vi "Error Query.vi"(8 "error in (no error)":errorcluster, 11 "VISA resource name":refnum<visa-resource-name>) -> (0 "error out":errorcluster, 1 "Error Message":string, 2 "error":bool, 3 "VISA resource name out":refnum<visa-resource-name>)   [LabVIEW 2020, in "Agilent 6XXX Series.lvlib"]
doc: "This VI reads an error from the instrument. It expects to see errors in SCPI format (#,\"error message\")."
uses:
  <instrlib>/Agilent 6XXX Series/Agilent 6XXX Series.lvlib
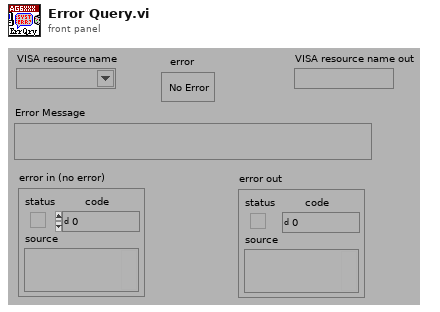
[diagram p1: front panel]
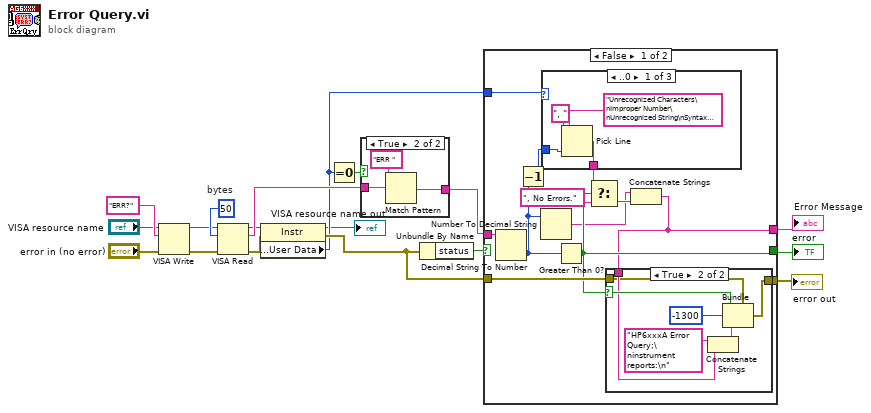
[diagram p0: block diagram]
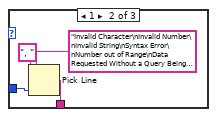
[diagram p3: hidden frame]
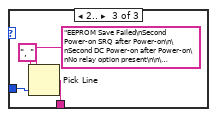
[diagram p4: hidden frame]
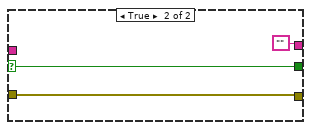
[diagram p6: hidden frame]
diagram:
  w15 = u32 50  # bytes
  n1 = VISA Write(VISA resource name="VISA resource name", write buffer="ERR?" ("error query command"), error in (no error)="error in (no error)") -> (VISA resource name out=w1:refnum<visa-resource-name>, error out=w2:errorcluster)  [unwired: 1 out]
  n2 = VISA Read(VISA resource name=w1, byte count=w15, error in (no error)=w2) -> (VISA resource name out=w4:refnum<visa-resource-name>, read buffer=w9:string, error out=w3:errorcluster)  [unwired: 1 out]
  n3 = property class="Instr"(reference=w4, error in=w3) -> (reference out=→"VISA resource name out":refnum<visa-resource-name>, error out=w7:errorcluster, "General Settings:User Data"=w6:u32)
  n4 = Equal To 0?(x=w6) -> (x = 0?=w10:bool)
  n5 = case shown="True" w10 {
    tunnel: w9 -> [w19 w22]
    tunnel: [w19 w21] -> w8
    frame False {
    }
    frame True {
      n6 = Match Pattern(string=w22, regular expression="ERR ") -> (after substring=w21:string)  [unwired: 1 in, 3 out]
    }
  }
  n7 = Unbundle By Name(w7) -> ("status"=w14:bool)
  n8 = case shown="False" w14 {
    selector: w14 -> [_ w56]
    tunnel: w8 -> [w28 _]
    tunnel: w7 -> [w34 w57]
    tunnel: [w33 w57] -> w11
    tunnel: [w32 w56] -> w13
    tunnel: [w29 ""] -> w12
    tunnel: w6 -> [w26 _]
    frame False {
      n9 = Decimal String To Number(string=w28) -> (number=w25:i32)  [unwired: 2 in, 1 out]
      n10 = Decrement(x=w25) -> (x-1=w23:i32)
      n11 = Number To Decimal String(number=w25) -> (decimal integer string=w27:string)  [unwired: 1 in]
      n12 = case shown="..0" w26 {
        tunnel: w23 -> [w37 w41 w45]
        tunnel: [w36 w40 w44] -> w24
        frame ..0 {
          n13 = Pick Line(string ("")=", ", multi-line string="Unrecognized Characters\nImproper Number\nUnrecognized String\nSyntax Error\nNumber out of Range\nAttempt to Exceed Soft Limits\nImproper Soft Limit\nData Requested Without a Query Being Sent\nRelay Error", line index=w37) -> (output string=w36:string)
        }
        frame 1 {
          n14 = Pick Line(string ("")=", ", multi-line string="Invalid Character\nInvalid Number\nInvalid String\nSyntax Error\nNumber out of Range\nData Requested Without a Query Being Sent\nString exceeds Display Length\nBuffer Full\nEEPROM Error\nHardware Error\nHardware Error - Channel 1\nHardware Error - Channel 2\nHardware Error - Channel 3\nHardware Error - Channel 4\nNo Model Number\nCalibration Error\nUncalibrated\nCalibration Locked\n\n\n\nSkip Self-Test\n\n\n\n\n\nInvalid String", line index=w41) -> (output string=w40:string)
        }
        frame 2.. {
          n15 = Pick Line(string ("")=", ", multi-line string="EEPROM Save Failed\nSecond Power-on SRQ after Power-on\n\nSecond DC Power-on after Power-on\nNo relay option present\n\n\nAddressed to talk and nothing to say\n\nHeader Expected\nUnrecognized Header\n\n\n\n\n\n\n\n\nNumber Expected\nNumber Syntax\nNumber out of Internal Range\n\n\n\n\n\n\n\nComma\nTerminator Expected\n\n\n\n\n\n\n\n\n\nParameter Out of Range\nVoltage Programming Error\nCurrent Programming Error\nOvervoltage Programming Error\nDelay Programming Error\nMask Programming Error\n\n\n\nMultiple CSAVE Commands\nEEPROM Checksum\nCalibration Mode Disabled\nCalibration Channel Out of Range\nCalibration Full Scale Out of Range\nCalibration Offset Out of Range\n\n\n\nCalibration Disable Jumper In", line index=w45) -> (output string=w44:string)
        }
      }
      n16 = Greater Than 0?(x=w25) -> (x > 0?=w32:bool)
      n17 = Select(t=w24, s=w32, f=", No Errors.") -> (s? t:f=w30:string)
      n18 = Concatenate Strings(w27, w30) -> (w29:string)
      n19 = case shown="True" w32 {
        selector: w32 -> [_ w51]
        tunnel: w29 -> [_ w50]
        tunnel: w34 -> [w47 w49]
        tunnel: [w47 w48] -> w33
        frame False {
        }
        frame True {
          n20 = Concatenate Strings("HP6xxxA Error Query;\ninstrument reports:\n", w50) -> (w52:string)
          n21 = Bundle(cluster=w49, "status"=w51, "code"=-1300, "source"=w52) -> (w48:errorcluster)
        }
      }
    }
    frame True {
    }
  }
  "Error Message" <- w12
  "error out" <- w11
  "error" <- w13
